vi "Configure Third Order Intercept (Zero Span Measurement).vi"(0 "VISA resource name":refnum<visa-resource-name>, 1 "TOI Resolution Bandwidth  (300:300Hz)":dbl(ring)=300.0 items=["30"=30.0, "100"=100.0, "300"=300.0, "1K"=1000.0, "3K"=3000.0, "10K"=10000.0, "30K"=30000.0, "100K"=100000.0, "300K"=300000.0, "1M"=1000000.0, "3M"=3000000.0, "50K"=50000.0, "5M"=5000000.0, "10M"=10000000.0, "20M"=20000000.0, "31.25M"=31250000.0], 2 "TOI Resolution Bandwidth Auto  (T:Enable)":bool=TRUE, 5 "TOI Sweep Time Auto  (T:Enable)":bool=TRUE, 7 "TOI Sweep Time (2s)":dbl=2.0 min=1e-06 max=1000.0, 9 "TOI Zero Span Measurement (1:On)":i32(ring)=1 items=["Off", "On"], 11 "error in (no error)":errorcluster) -> (4 "VISA resource name out":refnum<visa-resource-name>, 15 "error out":errorcluster)   [LabVIEW 2020, in "Anritsu Signal Analyzer Series.lvlib"]
doc: "Sets the parameter for zero span measurement of Spurious Emission measurement."
uses:
  Anritsu Signal Analyzer Series.lvlib
panel:
  # "Hz"
  # "s"
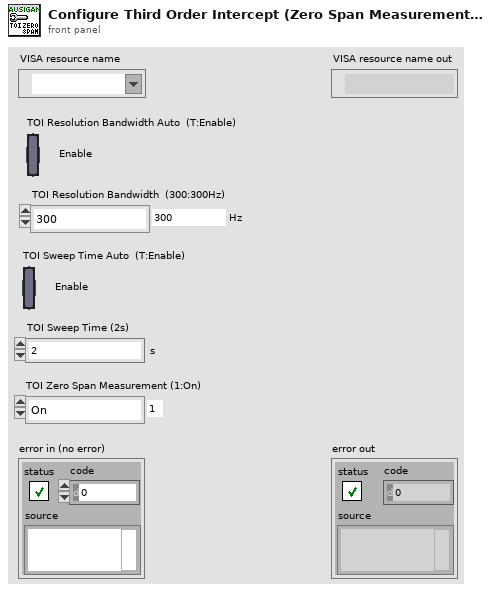
[diagram p1: front panel]
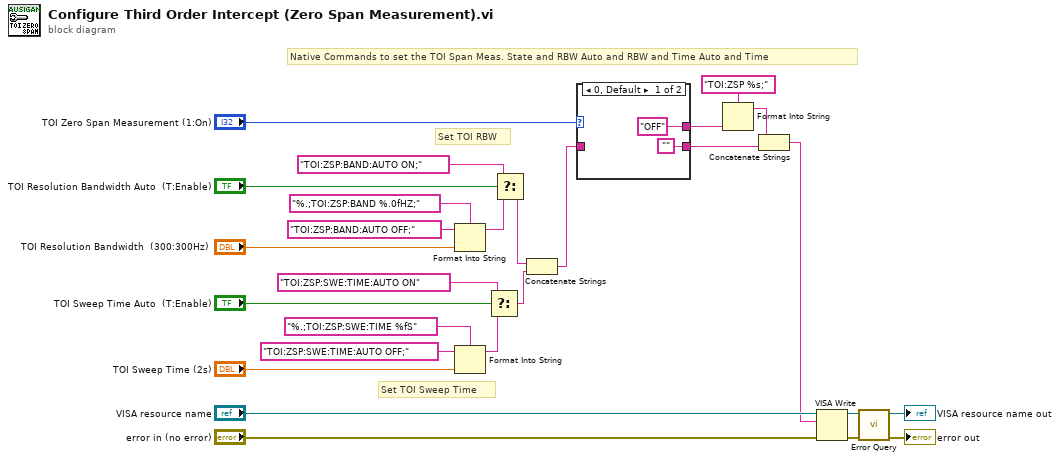
[diagram p0: block diagram]
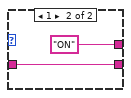
[diagram p2: hidden frame]
diagram:
  # "Native Commands to set the TOI Span Meas. State and RBW Auto and RBW and Time Auto and Time"
  # "Set TOI Sweep Time"
  # "Set TOI RBW"
  n1 = Format Into String(format string="%.;TOI:ZSP:BAND %.0fHZ;" ("Format String"), initial string="TOI:ZSP:BAND:AUTO OFF;" ("_CommandSet"), "TOI Resolution Bandwidth  (300:300Hz)") -> (resulting string=w3:string)  [unwired: 1 in, 1 out]
  n2 = Format Into String(format string="%.;TOI:ZSP:SWE:TIME %fS" ("Format String"), initial string="TOI:ZSP:SWE:TIME:AUTO OFF;" ("_CommandSet"), "TOI Sweep Time (2s)") -> (resulting string=w9:string)  [unwired: 1 in, 1 out]
  n3 = Select(t="TOI:ZSP:SWE:TIME:AUTO ON" ("_CommandSet"), s="TOI Sweep Time Auto  (T:Enable)", f=w9) -> (s? t:f=w8:string)
  n4 = Select(t="TOI:ZSP:BAND:AUTO ON;" ("_CommandSet"), s="TOI Resolution Bandwidth Auto  (T:Enable)", f=w3) -> (s? t:f=w2:string)
  n5 = Concatenate Strings(w2, w8) -> (w16:string)
  n6 = case shown="0, Default" "TOI Zero Span Measurement (1:On)" {
    tunnel: ["OFF" ("_Case1") "ON" ("_Case0")] -> w21
    tunnel: w16 -> [_ w30]
    tunnel: ["" w30] -> w15
    frame 0, Default {
    }
    frame 1 {
    }
  }
  n7 = Format Into String(format string="TOI:ZSP %s;" ("_CommandSet"), w21) -> (resulting string=w17:string)  [unwired: 2 in, 1 out]
  n8 = Concatenate Strings(w17, w15) -> (w14:string)
  n9 = VISA Write(VISA resource name="VISA resource name", write buffer=w14, error in (no error)="error in (no error)") -> (VISA resource name out=w18:refnum<visa-resource-name>, error out=w19:errorcluster)  [unwired: 1 out]
  n10 = call "Error Query.vi"("error in (no error)"=w19, "VISA resource name"=w18) -> ("error out"=→"error out":errorcluster, "VISA resource name out"=→"VISA resource name out":refnum<visa-resource-name>)  [unwired: 6 in, 2 out]
